vi "calc_phase_map2.vi"(4 "u8_ar_image_pixel_array":i16[][][](array[numeric])) -> (0 "raw phase map array":u8[][](array[numeric]))   [LabVIEW 2011]
panel:
  in  "add":dbl
  in  "multi":dbl
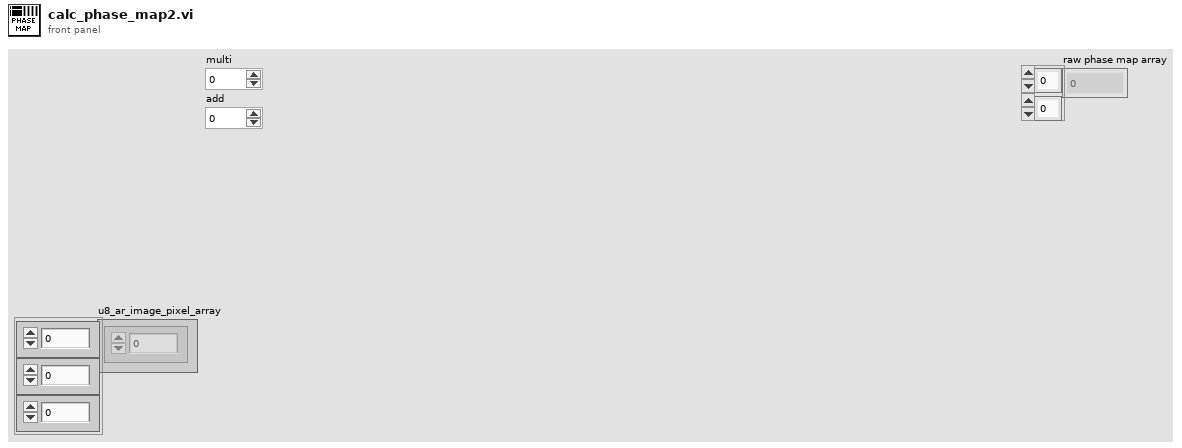
[diagram p1: front panel]
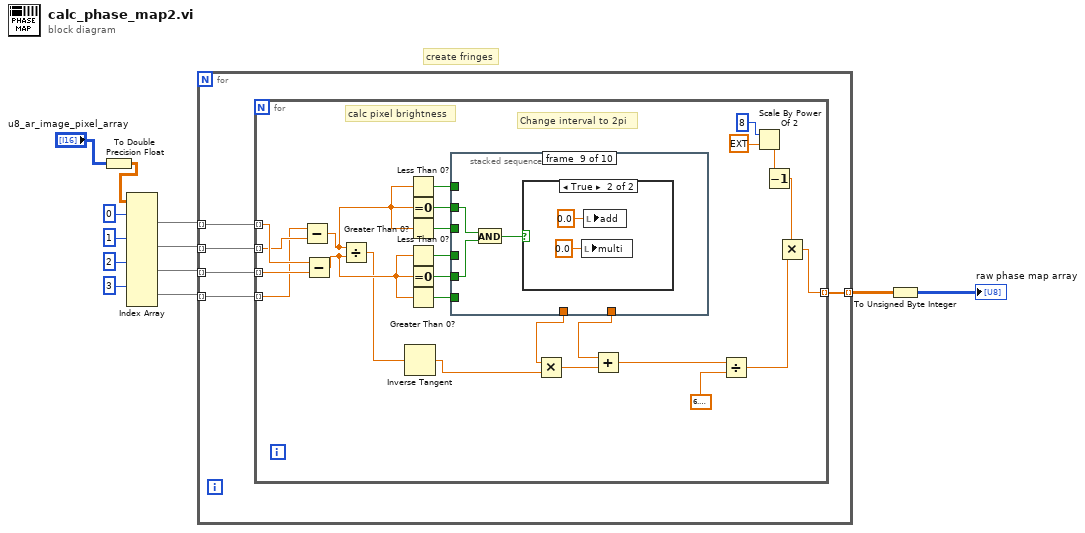
[diagram p0: block diagram]
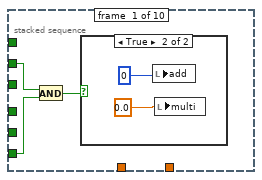
[diagram p2: hidden frame]
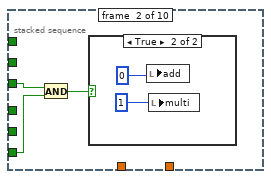
[diagram p4: hidden frame]
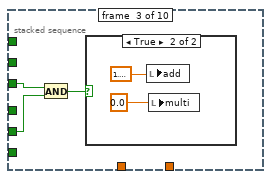
[diagram p6: hidden frame]
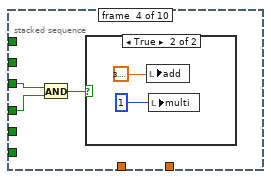
[diagram p8: hidden frame]
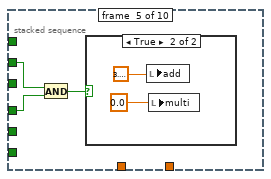
[diagram p10: hidden frame]
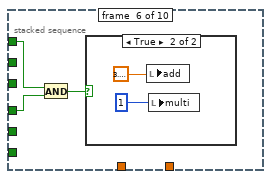
[diagram p12: hidden frame]
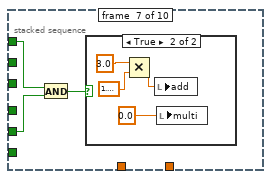
[diagram p14: hidden frame]
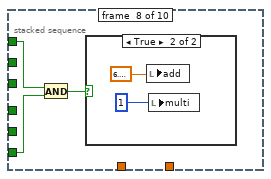
[diagram p16: hidden frame]
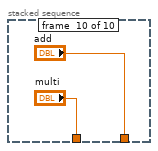
[diagram p19: hidden frame]
diagram:
  # "create fringes"
  n1 = To Double Precision Float(number="u8_ar_image_pixel_array") -> (double precision float=w1:dbl[][][])
  n2 = Index Array(array=w1, index (dim 0) #1=0 ("index (page)"), index (dim 0) #2=1 ("index (page)"), index (dim 0) #3=2 ("index (page)"), index (dim 0) #4=3 ("index (page)")) -> (element #1=w8:dbl[][], element #2=w7:dbl[][], element #3=w6:dbl[][], element #4=w5:dbl[][])  [unwired: 8 in]
  n3 = for {
    tunnel: w8 -> [w17] mode=indexing
    tunnel: w7 -> [w16] mode=indexing
    tunnel: w6 -> [w15] mode=indexing
    tunnel: w5 -> [w14] mode=indexing
    tunnel: [w13] -> w4 mode=indexing
    n4 = for {
      tunnel: w17 -> [w28] mode=indexing
      tunnel: w16 -> [w27] mode=indexing
      tunnel: w15 -> [w21] mode=indexing
      tunnel: w14 -> [w20] mode=indexing
      tunnel: [w38] -> w13 mode=indexing
      # "Change interval to 2pi"
      # "calc pixel brightness"
      n5 = Subtract(x=w20, y=w27) -> (x-y=w26:dbl)
      n6 = Subtract(x=w28, y=w21) -> (x-y=w25:dbl)
      n7 = Divide(x=w26, y=w25) -> (x/y=w19:dbl)
      n8 = Inverse Tangent(1:w19) -> (0:w18:dbl)
      n9 = Less Than 0?(x=w26) -> (x < 0?=w35:bool)
      n10 = Equal To 0?(x=w26) -> (x = 0?=w34:bool)
      n11 = Greater Than 0?(x=w26) -> (x > 0?=w33:bool)
      n12 = Less Than 0?(x=w25) -> (x < 0?=w30:bool)
      n13 = Equal To 0?(x=w25) -> (x = 0?=w31:bool)
      n14 = Greater Than 0?(x=w25) -> (x > 0?=w32:bool)
      n15 = stacked-sequence {
        tunnel: w35 -> [_ _ _ _ _ w69 w74 w80 _ _]
        tunnel: w34 -> [w44 _ _ _ w64 _ _ _ w85 _]
        tunnel: w33 -> [_ w49 w53 w59 _ _ _ _ _ _]
        tunnel: w32 -> [w43 w48 _ _ _ _ _ w81 _ _]
        tunnel: w31 -> [_ _ w54 _ _ _ w73 _ w86 _]
        tunnel: w30 -> [_ _ _ w58 w63 w68 _ _ _ _]
        tunnel: [_ _ _ _ _ _ _ _ _ "add"] -> w24
        tunnel: [_ _ _ _ _ _ _ _ _ "multi"] -> w22
        frame #0 {
          n16 = And(x=w44, y=w43) -> (x .and. y?=w45:bool)
          n17 = case shown="True" w45 {
            frame False {
            }
            frame True {
              n18 = local write "add"(0) -> ()
              n19 = local write "multi"(0.0) -> ()
            }
          }
        }
        frame #1 {
          n20 = And(x=w49, y=w48) -> (x .and. y?=w50:bool)
          n21 = case shown="True" w50 {
            frame False {
            }
            frame True {
              n22 = local write "add"(0) -> ()
              n23 = local write "multi"(1) -> ()
            }
          }
        }
        frame #2 {
          n24 = And(x=w53, y=w54) -> (x .and. y?=w55:bool)
          n25 = case shown="True" w55 {
            frame False {
            }
            frame True {
              n26 = local write "add"(1.5707963267948966) -> ()
              n27 = local write "multi"(0.0) -> ()
            }
          }
        }
        frame #3 {
          n28 = And(x=w59, y=w58) -> (x .and. y?=w60:bool)
          n29 = case shown="True" w60 {
            frame False {
            }
            frame True {
              n30 = local write "add"(3.141592653589793) -> ()
              n31 = local write "multi"(1) -> ()
            }
          }
        }
        frame #4 {
          n32 = And(x=w64, y=w63) -> (x .and. y?=w65:bool)
          n33 = case shown="True" w65 {
            frame False {
            }
            frame True {
              n34 = local write "add"(3.141592653589793) -> ()
              n35 = local write "multi"(0.0) -> ()
            }
          }
        }
        frame #5 {
          n36 = And(x=w69, y=w68) -> (x .and. y?=w70:bool)
          n37 = case shown="True" w70 {
            frame False {
            }
            frame True {
              n38 = local write "add"(3.141592653589793) -> ()
              n39 = local write "multi"(1) -> ()
            }
          }
        }
        frame #6 {
          n40 = And(x=w74, y=w73) -> (x .and. y?=w75:bool)
          n41 = case shown="True" w75 {
            frame False {
            }
            frame True {
              n42 = Multiply(x=3.0, y=1.5707963267948966) -> (x*y=w78:dbl)
              n43 = local write "add"(w78) -> ()
              n44 = local write "multi"(0.0) -> ()
            }
          }
        }
        frame #7 {
          n45 = And(x=w80, y=w81) -> (x .and. y?=w82:bool)
          n46 = case shown="True" w82 {
            frame False {
            }
            frame True {
              n47 = local write "add"(6.283185307179586) -> ()
              n48 = local write "multi"(1) -> ()
            }
          }
        }
        frame #8 {
          n49 = And(x=w85, y=w86) -> (x .and. y?=w87:bool)
          n50 = case shown="True" w87 {
            frame False {
            }
            frame True {
              n51 = local write "multi"(0.0 ("multi")) -> ()
              n52 = local write "add"(0.0 ("add")) -> ()
            }
          }
        }
        frame #9 {
        }
      }
      n53 = Multiply(x=w22, y=w18) -> (x*y=w23:dbl)
      n54 = Add(x=w24, y=w23) -> (x+y=w29:dbl)
      n55 = Divide(x=w29, y=6.283185307179586) -> (x/y=w39:dbl)
      n56 = Scale By Power Of 2(n=8, x=ext 1.0) -> (x*2^n=w41:ext)
      n57 = Decrement(x=w41) -> (x-1=w40:ext)
      n58 = Multiply(x=w40, y=w39) -> (x*y=w38:ext)
    }
  }
  n59 = To Unsigned Byte Integer(number=w4) -> (unsigned 8bit integer=→"raw phase map array":u8[][])
